vi "GPIBWaitForOperation.vi"(8 "error in (no error)":errorcluster, 11 "GPIB Address in":string) -> (0 "error out":errorcluster, 3 "GPIB Address out":string)   [LabVIEW 2017, in "LD Reading.lvclass"]
uses:
  LD Reading.lvclass
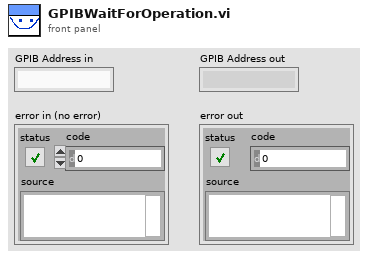
[diagram p1: front panel]
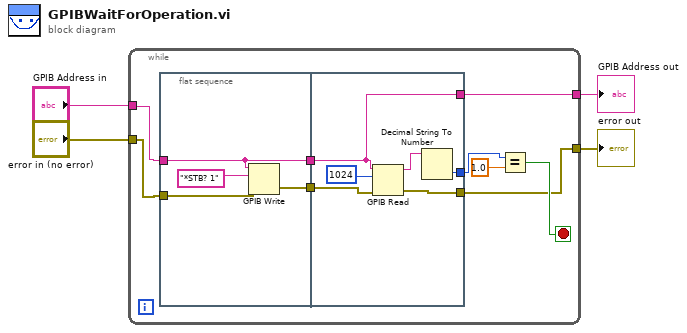
[diagram p0: block diagram]
diagram:
  n1 = while {
    tunnel: "GPIB Address in" -> [w8]
    tunnel: [w6] -> w2
    tunnel: "error in (no error)" -> [w7]
    tunnel: [w5] -> w4
    stop <- w10 stop-if-true
    n2 = flat-sequence {
      tunnel: w8 -> [w14]
      tunnel: [w16] -> w13
      tunnel: w7 -> [w15]
      tunnel: [w14] -> w9
      tunnel: [w22] -> w6
      tunnel: w13 -> [w21]
      tunnel: [w19] -> w11
      tunnel: w9 -> [w18]
      tunnel: [w18] -> w5
      frame #0 {
        n3 = GPIB Write(0:w14, 1:"*STB? 1" ("data"), 3:w15) -> (6:w16:errorcluster)  [unwired: 2 in, 1 out]
      }
      frame #1 {
        n4 = GPIB Read(0:w18, 1:1024 ("byte count"), 3:w21) -> (5:w20:string, 7:w22:errorcluster)  [unwired: 2 in, 1 out]
        n5 = Decimal String To Number(string=w20) -> (number=w19:i32)  [unwired: 2 in, 1 out]
      }
    }
    n6 = Equal?(x=w11, y=1.0) -> (x = y?=w10:bool)
  }
  "GPIB Address out" <- w4
  "error out" <- w2
